vi "Engine - Error - Error Logging.vi"(7 "Error Log FGV Cmd":T1(ring), 8 "error in (no error)":errorcluster) -> (0 "error out":errorcluster)   [LabVIEW 2015, in "DMM-SWITCH-ScanList Engine.lvlib"]
doc: "Error Loging Functional Global Variable\nSaves any errors in a text file in the Default Data Folder for the corresponding target"
uses:
  DMM-SWITCH-ScanList Engine.lvlib
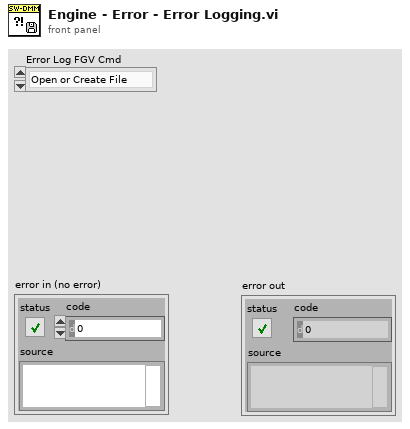
[diagram p1: front panel]
types:
  T1 = enum16{"Open or Create File", "Write Error", "Close File"}
  T2 = enum16{"open", "replace", "create", "open or create", "replace or create", "replace or create with confirmation"}
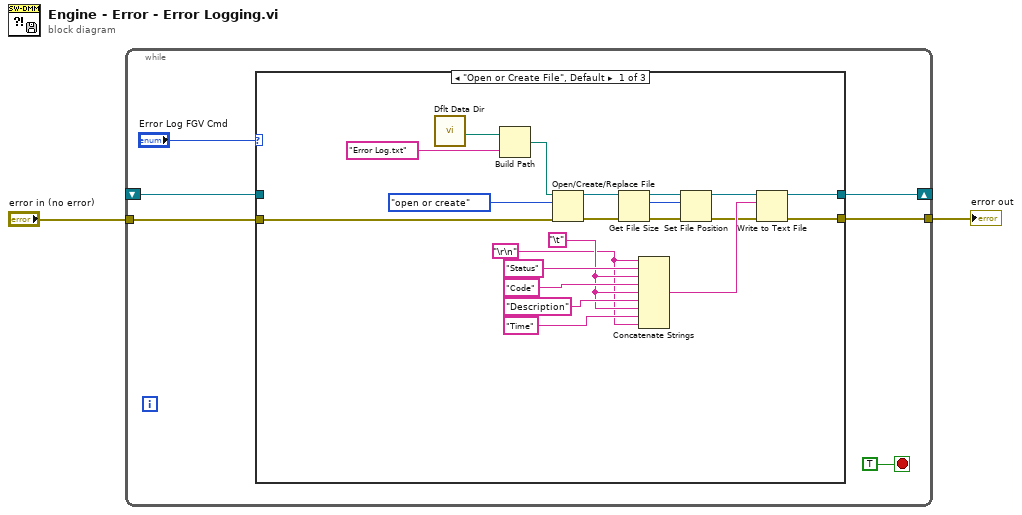
[diagram p0: block diagram]
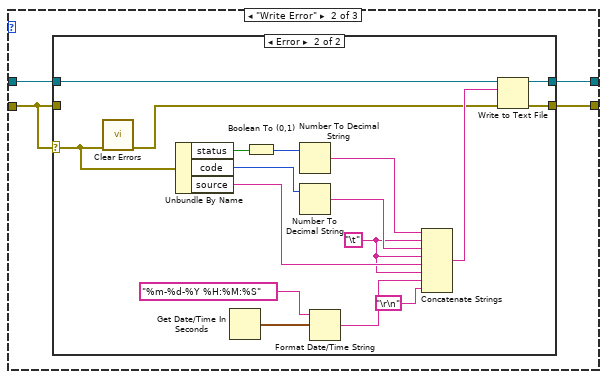
[diagram p2: hidden frame]
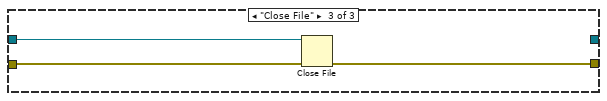
[diagram p4: hidden frame]
diagram:
  n1 = while {
    shift-right: [w8] -> _
    shift-left: _ -> [w7]
    tunnel: [w6] -> w1
    tunnel: "error in (no error)" -> [w3]
    stop <- TRUE stop-if-true
    n2 = case shown="\"Open or Create File\", Default" "Error Log FGV Cmd" {
      tunnel: [w16 w32 _] -> w8
      tunnel: w7 -> [_ w33 w55]
      tunnel: [w17 w31 w53] -> w6
      tunnel: w3 -> [w25 w30 w54]
      frame "Open or Create File", Default {
        w20 = "\t"
        w19 = "\r\n"
        n3 = call <vilib>:"Dflt Data Dir.vi"() -> ("App:Default Data Directory"=w28:path)
        n4 = Build Path(base path=w28, name or relative path="Error Log.txt") -> (appended path=w26:path)
        n5 = Open/Create/Replace File(file path (use dialog)=w26, error in=w25, operation (0:open)=T2."open or create") -> (refnum out=w15:refnum<file>, error out=w13:errorcluster)  [unwired: 3 in, 1 out]
        n6 = Get File Size(file=w15, error in=w13) -> (refnum out=w14:refnum<file>, size (in bytes)=w9:i64, 0:w11:errorcluster)
        n7 = Concatenate Strings(w19, "Status", w20, "Code", w20, "Description", w20, "Time", w19) -> (w18:string)
        n8 = Set File Position(offset (in bytes) (0)=w9, refnum=w14, error in=w11) -> (refnum out=w10:refnum<file>, error out=w12:errorcluster)  [unwired: 1 in]
        n9 = Write to Text File(file (use dialog)=w10, text=w18, error in=w12) -> (refnum out=w16:refnum<file>, error out=w17:errorcluster)  [unwired: 1 in, 1 out]
      }
      frame "Write Error" {
        n10 = case shown="Error" w30 {
          selector: w30 -> [_ w37]
          tunnel: w33 -> [w34 w52]
          tunnel: [w34 w51] -> w32
          tunnel: [w35 w50] -> w31
          tunnel: w30 -> [w35 _]
          frame No Error {
          }
          frame Error {
            w36 = "\t"
            n11 = call <vilib>:"Clear Errors.vi"("error in (no error)"=w37) -> ("error out"=w38:errorcluster)  [unwired: 5 in, 1 out]
            n12 = Unbundle By Name(w37) -> ("status"=w49:bool, "code"=w47:i32, "source"=w44:string)
            n13 = Get Date/Time In Seconds() -> (seconds since 1Jan1904=w42:timestamp)
            n14 = Boolean To (0,1)(Boolean=w49) -> (0, 1=w48:i16)
            n15 = Number To Decimal String(number=w48) -> (decimal integer string=w46:string)  [unwired: 1 in]
            n16 = Number To Decimal String(number=w47) -> (decimal integer string=w45:string)  [unwired: 1 in]
            n17 = Format Date/Time String(time format string (%c)="%m-%d-%Y %H:%M:%S", seconds (now)=w42) -> (date/time string=w40:string)  [unwired: 1 in]
            n18 = Concatenate Strings(w46, w36, w45, w36, w44, w36, w40, "\r\n") -> (w43:string)
            n19 = Write to Text File(file (use dialog)=w52, text=w43, error in=w38) -> (refnum out=w51:refnum<file>, error out=w50:errorcluster)  [unwired: 1 in, 1 out]
          }
        }
      }
      frame "Close File" {
        n20 = Close File(refnum=w55, error in=w54) -> (error out=w53:errorcluster)  [unwired: 1 out]
      }
    }
  }
  "error out" <- w1
